vi "Martinas Aging Program v1.0b.vi"() -> ()   [LabVIEW 2011]
uses:
  SubVIs/Control 3.ctl
  <vilib>/ULx/Create Channel.llb/ULx Create Channel (DO-Digital Output).vi
  <vilib>/ULx/Write.llb/ULx Write (Digital U32 1Chan 1Samp).vi
  C:/Program Files (x86)/National Instruments/LabVIEW 2009/instr.lib/Keithley 24XX/Keithley 24XX.lvlib
panel:
  out "Cell Settings Array":T1(array[cluster])=[{"Measure?"=TRUE, "Area (cm^2)"=0.0, "Cell Label"="", "Cell Description"="", "Time between scans (min)"=0.0, "Cell Position"=1, "Scan settings in queue"=0, "Sample holder"=1.0}, {"Measure?"=TRUE, "Area (cm^2)"=0.0, "Cell Label"="", "Cell Description"="", "Time between scans (min)"=0.0, "Cell Position"=2, "Scan settings in queue"=0, "Sample holder"=1.0}, {"Measure?"=TRUE, "Area (cm^2)"=0.0, "Cell Label"="", "Cell Description"="", "Time between scans (min)"=0.0, "Cell Position"=3, "Scan settings in queue"=0, "Sample holder"=1.0}, {"Measure?"=TRUE, "Area (cm^2)"=0.0, "Cell Label"="", "Cell Description"="", "Time between scans (min)"=0.0, "Cell Position"=4, "Scan settings in queue"=0, "Sample holder"=1.0}, {"Measure?"=TRUE, "Area (cm^2)"=0.0, "Cell Label"="", "Cell Description"="", "Time between scans (min)"=0.0, "Cell Position"=5, "Scan settings in queue"=0, "Sample holder"=1.0}, {"Measure?"=TRUE, "Area (cm^2)"=0.0, "Cell Label"="", "Cell Description"="", "Time between scans (min)"=0.0, "Cell Position"=6, "Scan settings in queue"=0, "Sample holder"=1.0}, {"Measure?"=TRUE, "Area (cm^2)"=0.0, "Cell Label"="", "Cell Description"="", "Time between scans (min)"=0.0, "Cell Position"=7, "Scan settings in queue"=0, "Sample holder"=1.0}, {"Measure?"=TRUE, "Area (cm^2)"=0.0, "Cell Label"="", "Cell Description"="", "Time between scans (min)"=0.0, "Cell Position"=8, "Scan settings in queue"=0, "Sample holder"=1.0}, {"Measure?"=TRUE, "Area (cm^2)"=0.0, "Cell Label"="", "Cell Description"="", "Time between scans (min)"=0.0, "Cell Position"=9, "Scan settings in queue"=0, "Sample holder"=1.0}, {"Measure?"=TRUE, "Area (cm^2)"=0.0, "Cell Label"="", "Cell Description"="", "Time between scans (min)"=0.0, "Cell Position"=10, "Scan settings in queue"=0, "Sample holder"=1.0}, {"Measure?"=TRUE, "Area (cm^2)"=0.0, "Cell Label"="", "Cell Description"="", "Time between scans (min)"=0.0, "Cell Position"=11, "Scan settings in queue"=0, "Sample holder"=1.0}, {"Measure?"=TRUE, "Area (cm^2)"=0.0, "Cell Label"="", "Cell Description"="", "Time between scans (min)"=0.0, "Cell Position"=12, "Scan settings in queue"=0, "Sample holder"=1.0}, {"Measure?"=TRUE, "Area (cm^2)"=0.0, "Cell Label"="", "Cell Description"="", "Time between scans (min)"=0.0, "Cell Position"=13, "Scan settings in queue"=0, "Sample holder"=1.0}, {"Measure?"=TRUE, "Area (cm^2)"=0.0, "Cell Label"="", "Cell Description"="", "Time between scans (min)"=0.0, "Cell Position"=14, "Scan settings in queue"=0, "Sample holder"=1.0}, {"Measure?"=TRUE, "Area (cm^2)"=0.0, "Cell Label"="", "Cell Description"="", "Time between scans (min)"=0.0, "Cell Position"=15, "Scan settings in queue"=0, "Sample holder"=1.0}, {"Measure?"=TRUE, "Area (cm^2)"=0.0, "Cell Label"="", "Cell Description"="", "Time between scans (min)"=0.0, "Cell Position"=16, "Scan settings in queue"=0, "Sample holder"=1.0}] {"Scan settings in queue" items=["Regular", "Inverted"]}
  in  "Port":refnum<k21>="Dev0/AuxPort"
  in  "VISA resource name":refnum<visa-resource-name>
  in  "Tab Control":T2(tab)
  in  "Cell Settings Array 1":T3(array[cluster])=[{"Measure?"=TRUE, "Area (cm^2)"=0.0, "Cell Label"="", "Cell Description"="", "Time between scans (s)"=0.0, "Cell Position"=1, "Scan settings in queue"=0, "Sample holder"=1.0}, {"Measure?"=TRUE, "Area (cm^2)"=0.0, "Cell Label"="", "Cell Description"="", "Time between scans (s)"=0.0, "Cell Position"=2, "Scan settings in queue"=0, "Sample holder"=1.0}, {"Measure?"=TRUE, "Area (cm^2)"=0.0, "Cell Label"="", "Cell Description"="", "Time between scans (s)"=0.0, "Cell Position"=3, "Scan settings in queue"=0, "Sample holder"=1.0}, {"Measure?"=TRUE, "Area (cm^2)"=0.0, "Cell Label"="", "Cell Description"="", "Time between scans (s)"=0.0, "Cell Position"=4, "Scan settings in queue"=0, "Sample holder"=1.0}, {"Measure?"=TRUE, "Area (cm^2)"=0.0, "Cell Label"="", "Cell Description"="", "Time between scans (s)"=0.0, "Cell Position"=5, "Scan settings in queue"=0, "Sample holder"=1.0}, {"Measure?"=TRUE, "Area (cm^2)"=0.0, "Cell Label"="", "Cell Description"="", "Time between scans (s)"=0.0, "Cell Position"=6, "Scan settings in queue"=0, "Sample holder"=1.0}, {"Measure?"=TRUE, "Area (cm^2)"=0.0, "Cell Label"="", "Cell Description"="", "Time between scans (s)"=0.0, "Cell Position"=7, "Scan settings in queue"=0, "Sample holder"=1.0}, {"Measure?"=TRUE, "Area (cm^2)"=0.0, "Cell Label"="", "Cell Description"="", "Time between scans (s)"=0.0, "Cell Position"=8, "Scan settings in queue"=0, "Sample holder"=1.0}, {"Measure?"=TRUE, "Area (cm^2)"=0.0, "Cell Label"="", "Cell Description"="", "Time between scans (s)"=0.0, "Cell Position"=9, "Scan settings in queue"=0, "Sample holder"=1.0}, {"Measure?"=TRUE, "Area (cm^2)"=0.0, "Cell Label"="", "Cell Description"="", "Time between scans (s)"=0.0, "Cell Position"=10, "Scan settings in queue"=0, "Sample holder"=1.0}, {"Measure?"=TRUE, "Area (cm^2)"=0.0, "Cell Label"="", "Cell Description"="", "Time between scans (s)"=0.0, "Cell Position"=11, "Scan settings in queue"=0, "Sample holder"=1.0}, {"Measure?"=TRUE, "Area (cm^2)"=0.0, "Cell Label"="", "Cell Description"="", "Time between scans (s)"=0.0, "Cell Position"=12, "Scan settings in queue"=0, "Sample holder"=1.0}, {"Measure?"=TRUE, "Area (cm^2)"=0.0, "Cell Label"="", "Cell Description"="", "Time between scans (s)"=0.0, "Cell Position"=13, "Scan settings in queue"=0, "Sample holder"=1.0}, {"Measure?"=TRUE, "Area (cm^2)"=0.0, "Cell Label"="", "Cell Description"="", "Time between scans (s)"=0.0, "Cell Position"=14, "Scan settings in queue"=0, "Sample holder"=1.0}, {"Measure?"=TRUE, "Area (cm^2)"=0.0, "Cell Label"="", "Cell Description"="", "Time between scans (s)"=0.0, "Cell Position"=15, "Scan settings in queue"=0, "Sample holder"=1.0}, {"Measure?"=TRUE, "Area (cm^2)"=0.0, "Cell Label"="", "Cell Description"="", "Time between scans (s)"=0.0, "Cell Position"=16, "Scan settings in queue"=0, "Sample holder"=1.0}] {"Scan settings in queue" items=["Regular", "Inverted"]}
  in  "Upload from Spreadsheet?":bool
  in  "Upload Spreadsheet path":path
  in  "Save to Spreadsheet?":bool
  in  "Save Spreadsheet Path":path
  in  "Cell Settings Array 2":T1(array[cluster])=[{"Measure?"=TRUE, "Area (cm^2)"=0.0, "Cell Label"="", "Cell Description"="", "Time between scans (min)"=0.0, "Cell Position"=1, "Scan settings in queue"=0, "Sample holder"=2.0}, {"Measure?"=TRUE, "Area (cm^2)"=0.0, "Cell Label"="", "Cell Description"="", "Time between scans (min)"=0.0, "Cell Position"=2, "Scan settings in queue"=0, "Sample holder"=2.0}, {"Measure?"=TRUE, "Area (cm^2)"=0.0, "Cell Label"="", "Cell Description"="", "Time between scans (min)"=0.0, "Cell Position"=3, "Scan settings in queue"=0, "Sample holder"=2.0}, {"Measure?"=TRUE, "Area (cm^2)"=0.0, "Cell Label"="", "Cell Description"="", "Time between scans (min)"=0.0, "Cell Position"=4, "Scan settings in queue"=0, "Sample holder"=2.0}, {"Measure?"=TRUE, "Area (cm^2)"=0.0, "Cell Label"="", "Cell Description"="", "Time between scans (min)"=0.0, "Cell Position"=5, "Scan settings in queue"=0, "Sample holder"=2.0}, {"Measure?"=TRUE, "Area (cm^2)"=0.0, "Cell Label"="", "Cell Description"="", "Time between scans (min)"=0.0, "Cell Position"=6, "Scan settings in queue"=0, "Sample holder"=2.0}, {"Measure?"=TRUE, "Area (cm^2)"=0.0, "Cell Label"="", "Cell Description"="", "Time between scans (min)"=0.0, "Cell Position"=7, "Scan settings in queue"=0, "Sample holder"=2.0}, {"Measure?"=TRUE, "Area (cm^2)"=0.0, "Cell Label"="", "Cell Description"="", "Time between scans (min)"=0.0, "Cell Position"=8, "Scan settings in queue"=0, "Sample holder"=2.0}, {"Measure?"=TRUE, "Area (cm^2)"=0.0, "Cell Label"="", "Cell Description"="", "Time between scans (min)"=0.0, "Cell Position"=9, "Scan settings in queue"=0, "Sample holder"=2.0}, {"Measure?"=TRUE, "Area (cm^2)"=0.0, "Cell Label"="", "Cell Description"="", "Time between scans (min)"=0.0, "Cell Position"=10, "Scan settings in queue"=0, "Sample holder"=2.0}, {"Measure?"=TRUE, "Area (cm^2)"=0.0, "Cell Label"="", "Cell Description"="", "Time between scans (min)"=0.0, "Cell Position"=11, "Scan settings in queue"=0, "Sample holder"=2.0}, {"Measure?"=TRUE, "Area (cm^2)"=0.0, "Cell Label"="", "Cell Description"="", "Time between scans (min)"=0.0, "Cell Position"=12, "Scan settings in queue"=0, "Sample holder"=2.0}, {"Measure?"=TRUE, "Area (cm^2)"=0.0, "Cell Label"="", "Cell Description"="", "Time between scans (min)"=0.0, "Cell Position"=13, "Scan settings in queue"=0, "Sample holder"=2.0}, {"Measure?"=TRUE, "Area (cm^2)"=0.0, "Cell Label"="", "Cell Description"="", "Time between scans (min)"=0.0, "Cell Position"=14, "Scan settings in queue"=0, "Sample holder"=2.0}, {"Measure?"=TRUE, "Area (cm^2)"=0.0, "Cell Label"="", "Cell Description"="", "Time between scans (min)"=0.0, "Cell Position"=15, "Scan settings in queue"=0, "Sample holder"=2.0}, {"Measure?"=TRUE, "Area (cm^2)"=0.0, "Cell Label"="", "Cell Description"="", "Time between scans (min)"=0.0, "Cell Position"=16, "Scan settings in queue"=0, "Sample holder"=2.0}] {"Scan settings in queue" items=["Regular", "Inverted"]}
  in  "Upload Spreadsheet path 2":path
  in  "Upload from Spreadsheet? 2":bool
  in  "Save Spreadsheet Path 2":path
  in  "Save to Spreadsheet?  2":bool
  in  "Cell Settings Array 3":T1(array[cluster])=[{"Measure?"=TRUE, "Area (cm^2)"=0.0, "Cell Label"="", "Cell Description"="", "Time between scans (min)"=0.0, "Cell Position"=1, "Scan settings in queue"=0, "Sample holder"=3.0}, {"Measure?"=TRUE, "Area (cm^2)"=0.0, "Cell Label"="", "Cell Description"="", "Time between scans (min)"=0.0, "Cell Position"=2, "Scan settings in queue"=0, "Sample holder"=3.0}, {"Measure?"=TRUE, "Area (cm^2)"=0.0, "Cell Label"="", "Cell Description"="", "Time between scans (min)"=0.0, "Cell Position"=3, "Scan settings in queue"=0, "Sample holder"=3.0}, {"Measure?"=TRUE, "Area (cm^2)"=0.0, "Cell Label"="", "Cell Description"="", "Time between scans (min)"=0.0, "Cell Position"=4, "Scan settings in queue"=0, "Sample holder"=3.0}, {"Measure?"=TRUE, "Area (cm^2)"=0.0, "Cell Label"="", "Cell Description"="", "Time between scans (min)"=0.0, "Cell Position"=5, "Scan settings in queue"=0, "Sample holder"=3.0}, {"Measure?"=TRUE, "Area (cm^2)"=0.0, "Cell Label"="", "Cell Description"="", "Time between scans (min)"=0.0, "Cell Position"=6, "Scan settings in queue"=0, "Sample holder"=3.0}, {"Measure?"=TRUE, "Area (cm^2)"=0.0, "Cell Label"="", "Cell Description"="", "Time between scans (min)"=0.0, "Cell Position"=7, "Scan settings in queue"=0, "Sample holder"=3.0}, {"Measure?"=TRUE, "Area (cm^2)"=0.0, "Cell Label"="", "Cell Description"="", "Time between scans (min)"=0.0, "Cell Position"=8, "Scan settings in queue"=0, "Sample holder"=3.0}, {"Measure?"=TRUE, "Area (cm^2)"=0.0, "Cell Label"="", "Cell Description"="", "Time between scans (min)"=0.0, "Cell Position"=9, "Scan settings in queue"=0, "Sample holder"=3.0}, {"Measure?"=TRUE, "Area (cm^2)"=0.0, "Cell Label"="", "Cell Description"="", "Time between scans (min)"=0.0, "Cell Position"=10, "Scan settings in queue"=0, "Sample holder"=3.0}, {"Measure?"=TRUE, "Area (cm^2)"=0.0, "Cell Label"="", "Cell Description"="", "Time between scans (min)"=0.0, "Cell Position"=11, "Scan settings in queue"=0, "Sample holder"=3.0}, {"Measure?"=TRUE, "Area (cm^2)"=0.0, "Cell Label"="", "Cell Description"="", "Time between scans (min)"=0.0, "Cell Position"=12, "Scan settings in queue"=0, "Sample holder"=3.0}, {"Measure?"=TRUE, "Area (cm^2)"=0.0, "Cell Label"="", "Cell Description"="", "Time between scans (min)"=0.0, "Cell Position"=13, "Scan settings in queue"=0, "Sample holder"=3.0}, {"Measure?"=TRUE, "Area (cm^2)"=0.0, "Cell Label"="", "Cell Description"="", "Time between scans (min)"=0.0, "Cell Position"=14, "Scan settings in queue"=0, "Sample holder"=3.0}, {"Measure?"=TRUE, "Area (cm^2)"=0.0, "Cell Label"="", "Cell Description"="", "Time between scans (min)"=0.0, "Cell Position"=15, "Scan settings in queue"=0, "Sample holder"=3.0}, {"Measure?"=TRUE, "Area (cm^2)"=0.0, "Cell Label"="", "Cell Description"="", "Time between scans (min)"=0.0, "Cell Position"=16, "Scan settings in queue"=0, "Sample holder"=3.0}] {"Scan settings in queue" items=["Regular", "Inverted"]}
  in  "Upload Spreadsheet path 3":path
  in  "Upload from Spreadsheet? 3":bool
  in  "Save Spreadsheet Path 3":path
  in  "Save to Spreadsheet?  3":bool
  in  "Cell Settings Array 4":T1(array[cluster])=[{"Measure?"=TRUE, "Area (cm^2)"=0.0, "Cell Label"="", "Cell Description"="", "Time between scans (min)"=0.0, "Cell Position"=1, "Scan settings in queue"=0, "Sample holder"=4.0}, {"Measure?"=TRUE, "Area (cm^2)"=0.0, "Cell Label"="", "Cell Description"="", "Time between scans (min)"=0.0, "Cell Position"=2, "Scan settings in queue"=0, "Sample holder"=4.0}, {"Measure?"=TRUE, "Area (cm^2)"=0.0, "Cell Label"="", "Cell Description"="", "Time between scans (min)"=0.0, "Cell Position"=3, "Scan settings in queue"=0, "Sample holder"=4.0}, {"Measure?"=TRUE, "Area (cm^2)"=0.0, "Cell Label"="", "Cell Description"="", "Time between scans (min)"=0.0, "Cell Position"=4, "Scan settings in queue"=0, "Sample holder"=4.0}, {"Measure?"=TRUE, "Area (cm^2)"=0.0, "Cell Label"="", "Cell Description"="", "Time between scans (min)"=0.0, "Cell Position"=5, "Scan settings in queue"=0, "Sample holder"=4.0}, {"Measure?"=TRUE, "Area (cm^2)"=0.0, "Cell Label"="", "Cell Description"="", "Time between scans (min)"=0.0, "Cell Position"=6, "Scan settings in queue"=0, "Sample holder"=4.0}, {"Measure?"=TRUE, "Area (cm^2)"=0.0, "Cell Label"="", "Cell Description"="", "Time between scans (min)"=0.0, "Cell Position"=7, "Scan settings in queue"=0, "Sample holder"=4.0}, {"Measure?"=TRUE, "Area (cm^2)"=0.0, "Cell Label"="", "Cell Description"="", "Time between scans (min)"=0.0, "Cell Position"=8, "Scan settings in queue"=0, "Sample holder"=4.0}, {"Measure?"=TRUE, "Area (cm^2)"=0.0, "Cell Label"="", "Cell Description"="", "Time between scans (min)"=0.0, "Cell Position"=9, "Scan settings in queue"=0, "Sample holder"=4.0}, {"Measure?"=TRUE, "Area (cm^2)"=0.0, "Cell Label"="", "Cell Description"="", "Time between scans (min)"=0.0, "Cell Position"=10, "Scan settings in queue"=0, "Sample holder"=4.0}, {"Measure?"=TRUE, "Area (cm^2)"=0.0, "Cell Label"="", "Cell Description"="", "Time between scans (min)"=0.0, "Cell Position"=11, "Scan settings in queue"=0, "Sample holder"=4.0}, {"Measure?"=TRUE, "Area (cm^2)"=0.0, "Cell Label"="", "Cell Description"="", "Time between scans (min)"=0.0, "Cell Position"=12, "Scan settings in queue"=0, "Sample holder"=4.0}, {"Measure?"=TRUE, "Area (cm^2)"=0.0, "Cell Label"="", "Cell Description"="", "Time between scans (min)"=0.0, "Cell Position"=13, "Scan settings in queue"=0, "Sample holder"=4.0}, {"Measure?"=TRUE, "Area (cm^2)"=0.0, "Cell Label"="", "Cell Description"="", "Time between scans (min)"=0.0, "Cell Position"=14, "Scan settings in queue"=0, "Sample holder"=4.0}, {"Measure?"=TRUE, "Area (cm^2)"=0.0, "Cell Label"="", "Cell Description"="", "Time between scans (min)"=0.0, "Cell Position"=15, "Scan settings in queue"=0, "Sample holder"=4.0}, {"Measure?"=TRUE, "Area (cm^2)"=0.0, "Cell Label"="", "Cell Description"="", "Time between scans (min)"=0.0, "Cell Position"=16, "Scan settings in queue"=0, "Sample holder"=4.0}] {"Scan settings in queue" items=["Regular", "Inverted"]}
  in  "Upload Spreadsheet path 4":path
  in  "Upload from Spreadsheet? 4":bool
  in  "Save Spreadsheet Path 4":path
  in  "Save to Spreadsheet?  4":bool
  out "Table":string[][](table)
  out "JV Curve":cluster{"Y":dbl[], "Y":dbl[]}[](graph)
  in  "Scan Switch":T4=TRUE
  in  "Stop Scan":T4=TRUE
  in  "Upload to the Queue":bool
  in  "Emergency Stop":bool
  in  "Scan settings":u16(ring) items=["Regular", "Inverted"]
  in  "Scan Settings JV":T5={"Light Intensity (Suns)"=1.0, "Stabilization Time (s)"=5.0, "Maximum Voltage (V)"=0.0, "Minimum Voltage (V)"=-1.0, "Range Options"=0, "Scan Direction\nDU (T), UD (F)"=TRUE, "Step Size (V)"=0.01, "Source Delay (s)"=0.15} {"Range Options" items=["Auto Range", "Semi-Auto Range", "100 uA", "1 mA", "10 mA", "100 mA", "1A"]}
  in  "Scan Setting Name":string
  in  "Add to Menu ring":bool
  out "Show me Scan \nSettings JV set":T5={"Light Intensity (Suns)"=1.0, "Stabilization Time (s)"=5.0, "Maximum Voltage (V)"=0.0, "Minimum Voltage (V)"=-1.0, "Range Options"=0, "Scan Direction\nDU (T), UD (F)"=TRUE, "Step Size (V)"=0.01, "Source Delay (s)"=0.15} {"Range Options" items=["Auto Range", "Semi-Auto Range", "100 uA", "1 mA", "10 mA", "100 mA", "1A"]}
  in  "Delete from Menu Ring":bool
  out "TIMER":dbl format="%<%H:%M:%S>t"
  in  "User Set?":bool
  in  "Logout":bool
  in  "Login":bool
  out "Username":string caption="Logged in as:"
  in  "Queue":T6(array[cluster]) {"Scan settings in queue" items=["Regular", "Inverted"]; "Time of the last scan (s)" format="%<%H:%M:%S>t"; "When did you stick it in?" format="%<%H:%M:%S>t"; "Time to next scan (s)" format="%<%H:%M:%S>t"; "Time in rig (s)" format="%<%H:%M:%S>t"}
  # "Area\n(cm^2)"
  # "Time between scans (s)"
  # "Time in rig\n(hrs)"
  # "Time since the last scan (hrs)"
  # "Scan\nnumber"
  # "When did you stick it in?"
  # "Time of the last scan"
  # "Sample\nHolder"
  # "On = working cell\nOff = not working cell"
  # "Label"
  # "Comment"
  # "Cell position"
  # "Scan Settings"
  # "Time between Scans (s)"
  # "Cell\nPosition"
  # "Sample\nHolder"
  # "On = working cell\nOff = not working cell"
  # "Area"
  # "Label"
  # "Comment"
  # "Scan Settings"
  # "Time between Scans (s)"
  # "Cell\nPosition"
  # "Sample\nHolder"
  # "On = working cell\nOff = not working cell"
  # "Area"
  # "Label"
  # "Comment"
  # "Scan Settings"
  # "Time between Scans (s)"
  # "Cell\nPosition"
  # "Sample\nHolder"
  # "On = working cell\nOff = not working cell"
  # "Area"
  # "Label"
  # "Comment"
  # "Scan Settings"
  # "Time between Scans (s)"
  # "Cell\nPosition"
  # "Sample\nHolder"
  # "On = working cell\nOff = not working cell"
  # "Area"
  # "Label"
  # "Comment"
  # "Scan Settings"
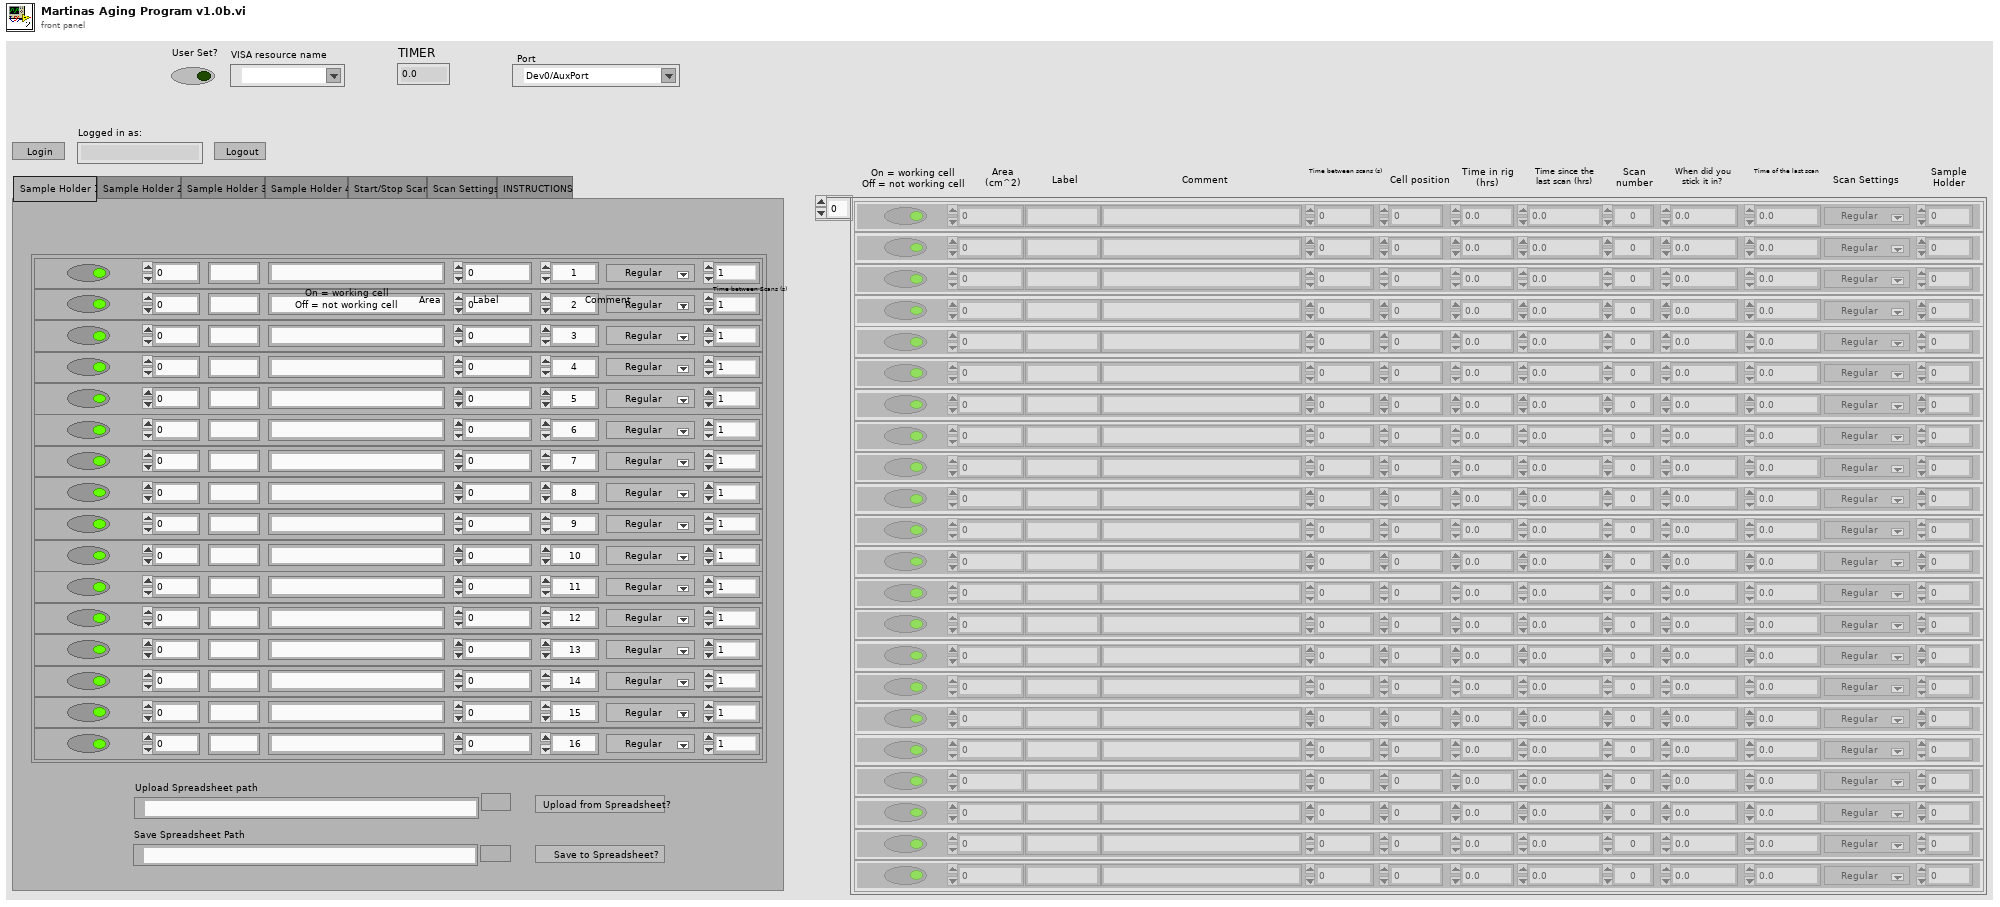
[diagram p1: front panel]
types:
  T1 = cluster{"Measure?":bool, "Area (cm^2)":dbl, "Cell Label":string, "Cell Description":string, "Time between scans (min)":dbl, "Cell Position":i32, "Scan settings in queue":u16, "Sample holder":dbl}[]
  T2 = enum32{"Sample Holder 1", "Sample Holder 2", "Sample Holder 3", "Sample Holder 4", "Start/Stop Scan", "Scan Settings", "INSTRUCTIONS"}
  T3 = cluster{"Measure?":bool, "Area (cm^2)":dbl, "Cell Label":string, "Cell Description":string, "Time between scans (s)":dbl, "Cell Position":i32, "Scan settings in queue":u16, "Sample holder":dbl}[]
  T4 = typedef "Control 3.ctl" = bool
  T5 = cluster{"Light Intensity (Suns)":dbl, "Stabilization Time (s)":dbl, "Maximum Voltage (V)":dbl, "Minimum Voltage (V)":dbl, "Range Options":u16, "Scan Direction\nDU (T), UD (F)":bool, "Step Size (V)":dbl, "Source Delay (s)":dbl}
  T6 = cluster{"Measure?":bool, "Area (cm^2)":dbl, "Cell Label":string, "Cell Description":string, "Cell Position":i32, "Time in rig (s)":dbl, "Time to next scan (s)":dbl, "Scan number":dbl, "When did you stick it in?":dbl, "Time between scans (s)":dbl, "Time of the last scan (s)":dbl, "Scan settings in queue":u16, "Sample Holder":dbl}[]
  T7 = enum8{"Enabled", "Disabled", "Disabled and Grayed Out"}
  T8 = cluster{"Light Intensity (Suns)":dbl, "Stabilization Time (s)":dbl, "Maximum Voltage (V)":dbl, "Minimum Voltage (V)":dbl, "Range Options":u16, "Scan Direction\nDU (T), UD (F)":bool, "Step Size (V)":dbl, "Source Delay (s)":dbl}[]
  T9 = cluster{"Measure?":bool, "Area (cm^2)":dbl, "Cell Label":string, "Cell Description":string, "Cell Position":i32, "Time in rig (s)":dbl, "Time to next scan (s)":dbl, "Scan number":dbl, "When did you stick it in?":dbl, "Time between scans (s)":dbl, "Time of the last scan (s)":dbl, "Scan settings in queue":u16, "Sample Holder":dbl}
  T10 = typedef "imagedata.ctl" = cluster{"image type":i32, "image depth":i32, "image":u8[], "mask":u8[], "colors":u32[], "Rectangle":cluster{"left":i16, "top":i16, "right":i16, "bottom":i16}}
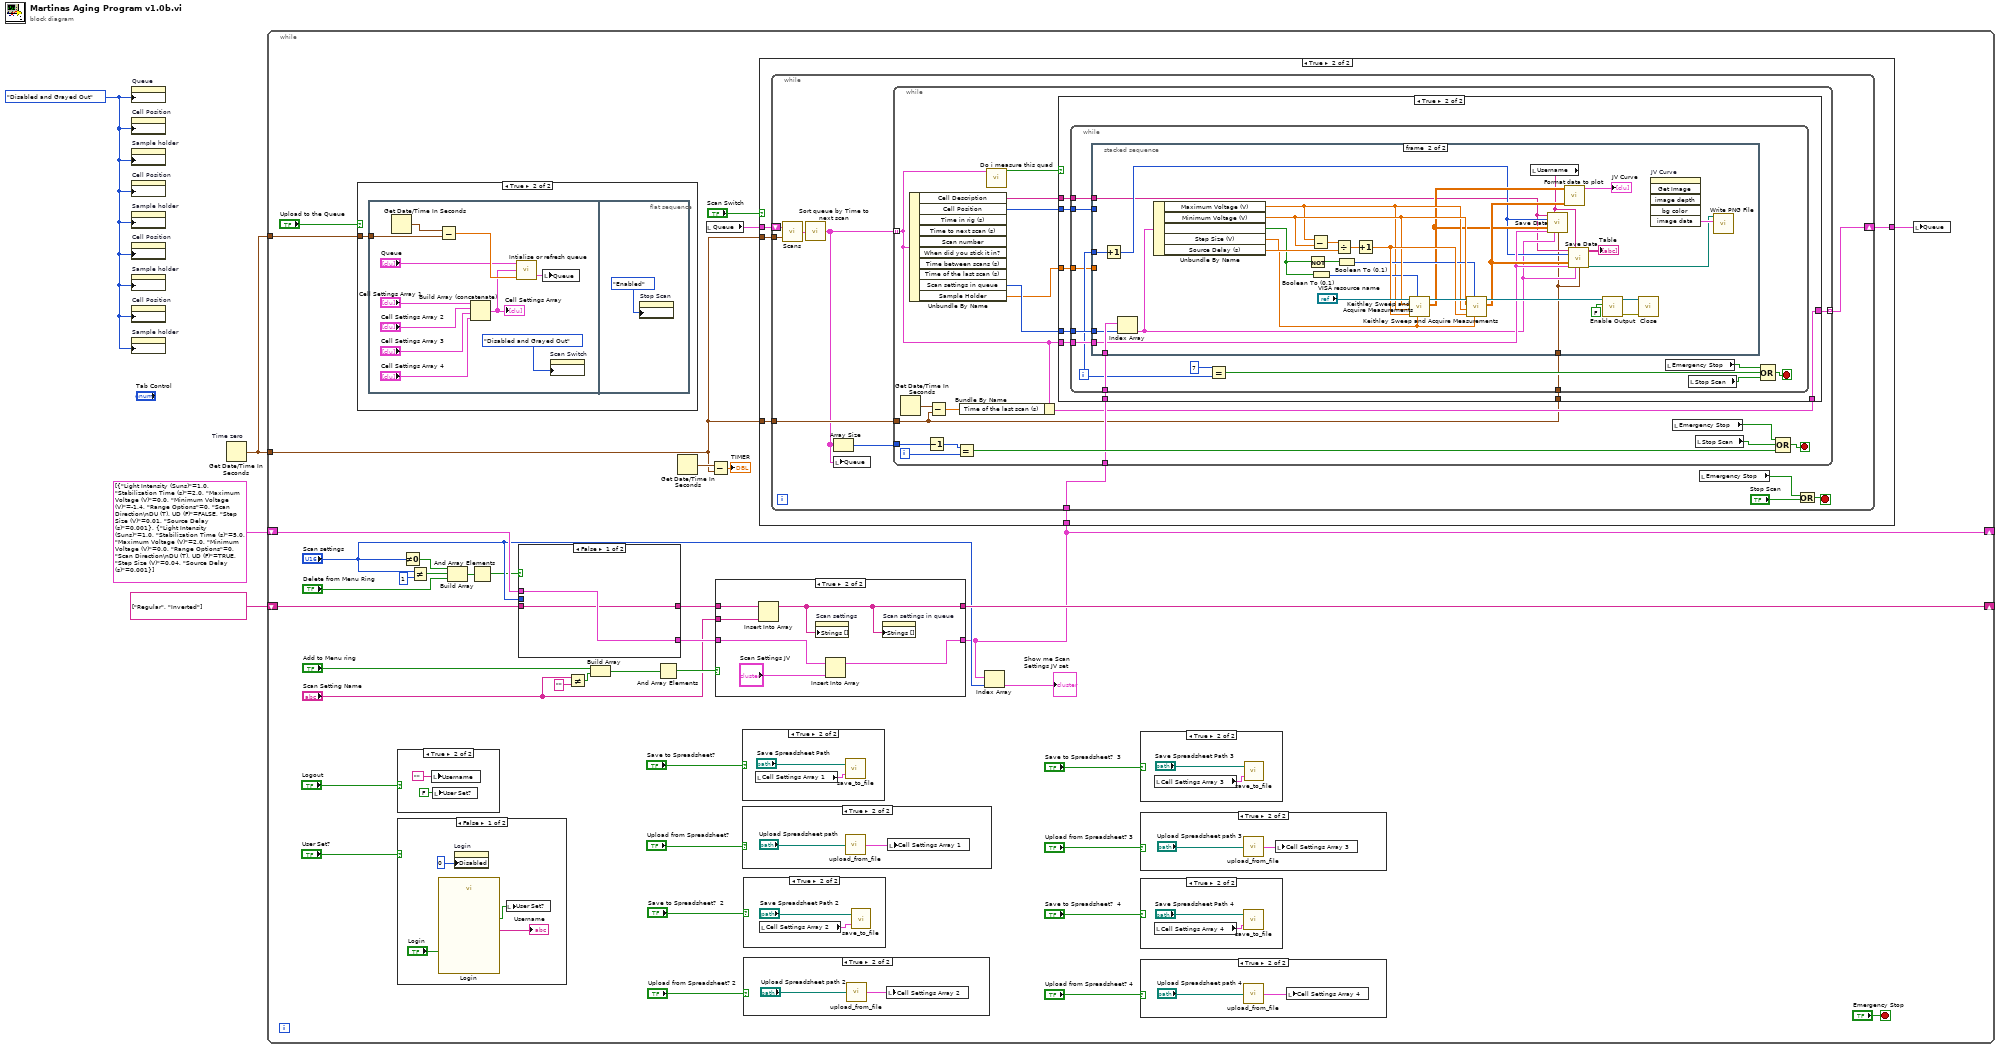
[diagram p0: block diagram]
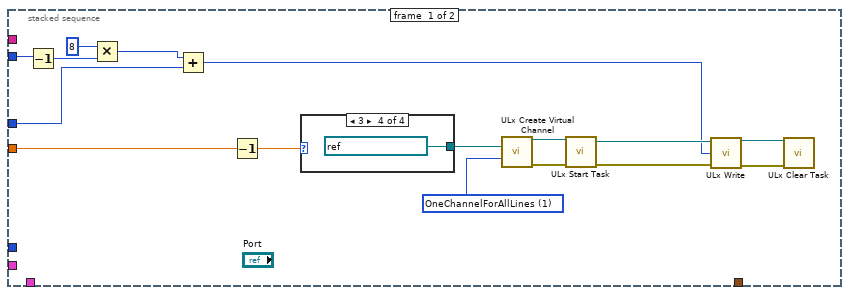
[diagram p10: hidden frame]
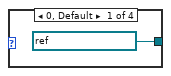
[diagram p11: hidden frame]
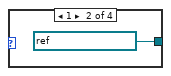
[diagram p12: hidden frame]
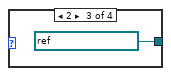
[diagram p13: hidden frame]
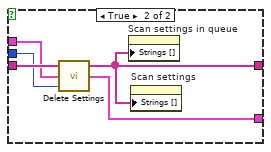
[diagram p14: hidden frame]
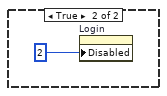
[diagram p17: hidden frame]
diagram:
  w1 = T7."Disabled and Grayed Out" ("Disabled")
  n1 = property on="Queue" class="Arr (strict)"("DisabledEnum"=w1) -> ()  [unwired: 2 in, 2 out]
  n2 = property on="Cell Position" class="DigNum (strict)"("DisabledEnum"=w1) -> ()  [unwired: 2 in, 2 out]
  n3 = property on="Sample holder" class="DigNum (strict)"("DisabledEnum"=w1) -> ()  [unwired: 2 in, 2 out]
  n4 = property on="Cell Position" class="DigNum (strict)"("DisabledEnum"=w1) -> ()  [unwired: 2 in, 2 out]
  n5 = property on="Sample holder" class="DigNum (strict)"("DisabledEnum"=w1) -> ()  [unwired: 2 in, 2 out]
  n6 = property on="Cell Position" class="DigNum (strict)"("DisabledEnum"=w1) -> ()  [unwired: 2 in, 2 out]
  n7 = property on="Sample holder" class="DigNum (strict)"("DisabledEnum"=w1) -> ()  [unwired: 2 in, 2 out]
  n8 = property on="Cell Position" class="DigNum (strict)"("DisabledEnum"=w1) -> ()  [unwired: 2 in, 2 out]
  n9 = property on="Sample holder" class="DigNum (strict)"("DisabledEnum"=w1) -> ()  [unwired: 2 in, 2 out]
  n10 = Get Date/Time In Seconds "Time zero"() -> (seconds since 1Jan1904=w2:timestamp)
  n11 = while {
    tunnel: w2 -> [w40]
    shift-right: [w7] -> _
    shift-left: T8 [{"Light Intensity (Suns)"=1.0, "Stabilization Time (s)"=2.0, "Maximum Voltage (V)"=0.0, "Minimum Voltage (V)"=-1.4, "Range Options"=0, "Scan Direction\nDU (T), UD (F)"=FALSE, "Step Size (V)"=0.01, "Source Delay (s)"=0.001}, {"Light Intensity (Suns)"=1.0, "Stabilization Time (s)"=5.0, "Maximum Voltage (V)"=2.0, "Minimum Voltage (V)"=0.0, "Range Options"=0, "Scan Direction\nDU (T), UD (F)"=TRUE, "Step Size (V)"=0.04, "Source Delay (s)"=0.001}] ("JV curve scan settings 2") -> [w34]
    shift-right: [w38] -> _
    shift-left: string[] ["Regular", "Inverted"] ("Strings []") -> [w35]
    tunnel: w2 -> [w6]
    stop <- "Emergency Stop" stop-if-true
    n12 = case shown="True" "Upload to the Queue" {
      tunnel: w40 -> [_ w188]
      frame False {
      }
      frame True {
        n13 = flat-sequence {
          tunnel: w188 -> [w199]
          frame #0 {
            n14 = Get Date/Time In Seconds() -> (seconds since 1Jan1904=w198:timestamp)
            n15 = Subtract(x=w198, y=w199) -> (x-y=w197:dbl)
            n16 = Build Array (concatenate)("Cell Settings Array 1", "Cell Settings Array 2", "Cell Settings Array 3", "Cell Settings Array 4") -> (w190:T1)
            "Cell Settings Array" <- w190
            n17 = call "Intialise or refresh queue.vi"("When did you stick it in?"=w197, "Cell Settings Array"=w190, "Queue in"="Queue") -> ("Queue out"=w196:T6)  [unwired: 1 in]
            n18 = local write "Queue"(w196) -> ()
            n19 = property on="Scan Switch" class="Bool (strict)"("DisabledEnum"=T7."Disabled and Grayed Out" ("Disabled")) -> ()  [unwired: 2 in, 2 out]
          }
          frame #1 {
            n20 = property on="Stop Scan" class="Bool (strict)"("DisabledEnum"=T7."Enabled" ("Disabled")) -> ()  [unwired: 2 in, 2 out]
          }
        }
      }
    }
    n21 = case shown="True" "Logout" {
      frame False {
      }
      frame True {
        n22 = local write "Username"("") -> ()
        n23 = local write "User Set?"(FALSE) -> ()
      }
    }
    n24 = case shown="False" "User Set?" {
      frame False {
        n25 = call "Login"("Enable"="Login") -> ("Username"=→"Username":string, "OK"=w183:bool)  [unwired: 16 in, 1 out]
        n26 = property on="Login" class="Bool"("Disabled"=0) -> ()  [unwired: 2 in, 2 out]
        n27 = local write "User Set?"(w183) -> ()
      }
      frame True {
        n28 = property on="Login" class="Bool"("Disabled"=2) -> ()  [unwired: 2 in, 2 out]
      }
    }
    n29 = Not Equal To 0?(x="Scan settings") -> (x != 0?=w31:bool)
    n30 = Not Equal?(x="Scan settings", y=u16 1) -> (x != y?=w28:bool)
    n31 = Build Array(w31, w28, "Delete from Menu Ring") -> (w26:bool[])
    n32 = And Array Elements(Boolean array=w26) -> (logical AND=w25:bool)
    n33 = case shown="False" w25 {
      tunnel: w35 -> [w166 w172]
      tunnel: w34 -> [w167 w171]
      tunnel: "Scan settings" -> [_ w170]
      tunnel: [w166 w169] -> w33
      tunnel: [w167 w168] -> w32
      frame False {
      }
      frame True {
        n34 = call "Delete Settings.vi"("Scan settings"=w170, "JV curve scan settings"=w171, "Strings In"=w172) -> ("JV curve scan settings Out"=w168:T8, "Strings Out"=w169:string[])  [unwired: 1 out]
        n35 = property on="Scan settings in queue" class="Ring (strict)"("Strings []"=w169) -> ()  [unwired: 2 in, 2 out]
        n36 = property on="Scan settings" class="Ring (strict)"("Strings []"=w169) -> ()  [unwired: 2 in, 2 out]
      }
    }
    n37 = Not Equal?(x="Scan Setting Name", y="") -> (x != y?=w22:bool)
    n38 = Build Array("Add to Menu ring", w22) -> (w23:bool[])
    n39 = And Array Elements(Boolean array=w23) -> (logical AND=w20:bool)
    n40 = Get Date/Time In Seconds() -> (seconds since 1Jan1904=w17:timestamp)
    n41 = local read "Queue"() -> (w15:T6)
    n42 = Subtract(x=w17, y=w6) -> (x-y=→"TIMER":dbl)
    n43 = case shown="True" w20 {
      tunnel: w32 -> [w174 w180]
      tunnel: [w174 w179] -> w7
      tunnel: w33 -> [w173 w176]
      tunnel: [w173 w177] -> w38
      tunnel: "Scan Setting Name" -> [_ w175]
      frame False {
      }
      frame True {
        n44 = Insert Into Array(array=w176, new element=w175) -> (w177:string[])  [unwired: 1 in]
        n45 = property on="Scan settings" class="Ring (strict)"("Strings []"=w177) -> ()  [unwired: 2 in, 2 out]
        n46 = Insert Into Array(array=w180, new element="Scan Settings JV") -> (w179:T8)  [unwired: 1 in]
        n47 = property on="Scan settings in queue" class="Ring (strict)"("Strings []"=w177) -> ()  [unwired: 2 in, 2 out]
      }
    }
    n48 = case shown="True" "Save to Spreadsheet?" {
      frame False {
      }
      frame True {
        n49 = local read "Cell Settings Array 1"() -> (w201:T3)
        n50 = call "save_to_file.vi"("Cell Settings Array 4"=w201, "Save Path"="Save Spreadsheet Path") -> ()  [unwired: 1 in]
      }
    }
    n51 = case shown="True" "Upload from Spreadsheet?" {
      frame False {
      }
      frame True {
        n52 = call "upload_from_file.vi"("Spreadsheet path"="Upload Spreadsheet path") -> ("Cell Settings Array 4"=w203:T1)
        n53 = local write "Cell Settings Array 1"(w203) -> ()
      }
    }
    n54 = case shown="True" "Save to Spreadsheet?  2" {
      frame False {
      }
      frame True {
        n55 = local read "Cell Settings Array 2"() -> (w52:T1)
        n56 = call "save_to_file.vi"("Cell Settings Array 4"=w52, "Save Path"="Save Spreadsheet Path 2") -> ()  [unwired: 1 in]
      }
    }
    n57 = case shown="True" "Upload from Spreadsheet? 2" {
      frame False {
      }
      frame True {
        n58 = call "upload_from_file.vi"("Spreadsheet path"="Upload Spreadsheet path 2") -> ("Cell Settings Array 4"=w54:T1)
        n59 = local write "Cell Settings Array 2"(w54) -> ()
      }
    }
    n60 = case shown="True" "Scan Switch" {
      tunnel: w15 -> [w56 w61]
      tunnel: w6 -> [_ w60]
      tunnel: [w56 w58] -> w5
      tunnel: w7 -> [_ w59]
      tunnel: w6 -> [_ w57]
      frame False {
      }
      frame True {
        n61 = while {
          tunnel: w60 -> [w71]
          tunnel: w59 -> [w69]
          shift-right: [w67] -> w58
          shift-left: w61 -> [w72]
          tunnel: w57 -> [w66]
          stop <- w64 stop-if-true
          n62 = call "Scans.vi"("Time zero (sec)"=w71, "Queue in"=w72) -> ("Queue out"=w70:T6)
          n63 = call "Sort queue by Time to next scan.vi"("Queue"=w70) -> ("Queue Out"=w65:T6)  [unwired: 4 in]
          n64 = Array Size(array=w65) -> (size(s)=w68:i32)
          n65 = local write "Queue"(w65) -> ()
          n66 = while {
            tunnel: w65 -> [w76] mode=indexing
            tunnel: w69 -> [w82]
            tunnel: w68 -> [w88]
            tunnel: [w83] -> w67 mode=indexing
            tunnel: w66 -> [w74]
            i -> [w90]
            stop <- w86 stop-if-true
            n67 = Get Date/Time In Seconds() -> (seconds since 1Jan1904=w78:timestamp)
            n68 = Unbundle By Name(w76) -> ("Cell Description"=w80:string, "Cell Position"=w84:i32, "Scan settings in queue"=w91:u16, "Sample Holder"=w81:dbl)  [unwired: 6 out]
            n69 = Decrement(x=w88) -> (x-1=w89:i32)
            n70 = Subtract(x=w78, y=w74) -> (x-y=w77:dbl)
            n71 = Equal?(x=w89, y=w90) -> (x = y?=w87:bool)
            n72 = Bundle By Name(cluster=w76, "Time of the last scan (s)"=w77) -> (w75:T9)
            n73 = call "Do i measure this quad.vi"("Cell details"=w76) -> ("Measure cell?"=w79:bool)  [unwired: 10 in]
            n74 = case shown="True" w79 {
              tunnel: w82 -> [_ w100]
              tunnel: w91 -> [_ w99]
              tunnel: w76 -> [w92 w98]
              tunnel: w84 -> [_ w97]
              tunnel: [w92 w94] -> w83
              tunnel: w81 -> [_ w96]
              tunnel: w80 -> [_ w95]
              tunnel: w75 -> [_ w94]
              tunnel: w74 -> [_ w93]
              frame False {
              }
              frame True {
                n75 = while {
                  tunnel: w100 -> [w113]
                  tunnel: w99 -> [w112]
                  tunnel: w98 -> [w111]
                  tunnel: w97 -> [w110]
                  tunnel: w96 -> [w104]
                  tunnel: w95 -> [w103]
                  tunnel: w93 -> [w102]
                  i -> [w105]
                  stop <- w107 stop-if-true
                  n76 = stacked-sequence {
                    tunnel: w113 -> [_ w161]
                    tunnel: w112 -> [_ w160]
                    tunnel: w111 -> [_ w141]
                    tunnel: w110 -> [w118 _]
                    tunnel: w105 -> [w115 w139]
                    tunnel: w104 -> [w114 _]
                    tunnel: w103 -> [_ w135]
                    tunnel: w102 -> [_ w134]
                    frame #0 {
                      w127 = 1 items=["OneChannelForEachLine", "OneChannelForAllLines"] ("line grouping")
                      n77 = Decrement(x=w118) -> (x-1=w117:i32)
                      n78 = Multiply(x=8, y=w117) -> (x*y=w119:i32)
                      n79 = Add(x=w119, y=w115) -> (x+y=w116:i32)
                      n80 = Decrement(x=w114) -> (x-1=w128:dbl)
                      n81 = case shown="3" w128 {
                        tunnel: [refnum<k21> "Dev0/1stPortA" ("Port 2") refnum<k21> "Dev0/1stPortB" ("Port 2") refnum<k21> "Dev0/1stPortA" ("Port 2") refnum<k21> "Dev0/1stPortB" ("Port 2")] -> w129
                        frame 0, Default {
                        }
                        frame 1 {
                        }
                        frame 2 {
                        }
                        frame 3 {
                        }
                      }
                      n82 = call-poly <vilib>:"ULx Create Virtual Channel.vi"("lines"=w129, "line grouping"=w127) -> ("task out"=w125:refnum<k24>, "error out"=w126:errorcluster)  [unwired: 12 in]
                      n83 = call <vilib>:"ULx Start Task.vi"("task in"=w125, "error in"=w126) -> ("task out"=w122:refnum<k24>, "error out"=w121:errorcluster)  [unwired: 12 in]
                      n84 = call-poly <vilib>:"ULx Write.vi"("task in"=w122, "data"=w116, "error in"=w121) -> ("task out"=w124:refnum<k24>, "error out"=w123:errorcluster)  [unwired: 10 in, 1 out]
                      n85 = call <vilib>:"ULx Clear Task.vi"("task in"=w124, "error in"=w123) -> ()  [unwired: 13 in, 1 out]
                    }
                    frame #1 {
                      n86 = Increment(x=w139) -> (x+1=w138:i32)
                      n87 = Index Array(array=w161, index=w160) -> (element=w137:T5)
                      n88 = Unbundle By Name(w137) -> ("Maximum Voltage (V)"=w147:dbl, "Minimum Voltage (V)"=w153:dbl, "Scan Direction\nDU (T), UD (F)"=w151:bool, "Step Size (V)"=w157:dbl, "Source Delay (s)"=w148:dbl)
                      n89 = Not(x=w151) -> (.not. x?=w152:bool)
                      n90 = Subtract(x=w147, y=w153) -> (x-y=w158:dbl)
                      n91 = Boolean To (0,1)(Boolean=w151) -> (0, 1=w149:i16)
                      n92 = Divide(x=w158, y=w157) -> (x/y=w159:dbl)
                      n93 = Boolean To (0,1)(Boolean=w152) -> (0, 1=w150:i16)
                      n94 = Increment(x=w159) -> (x+1=w155:dbl)
                      n95 = call "Keithley Sweep and Acquire Measurements.vi"("Source Delay (s)"=w148, "Sweep Direction"=w149, "Number of Points"=w155, "Maximum Amplitude"=w147, "Minimum Amplitude"=w153, "VISA resource name"="VISA resource name") -> ("Data Array"=w140:dbl[][], "VISA resource name out"=w156:refnum<visa-resource-name>)  [unwired: 1 in, 1 out]
                      n96 = call "Keithley Sweep and Acquire Measurements.vi"("Source Delay (s)"=w148, "Sweep Direction"=w150, "Number of Points"=w155, "Maximum Amplitude"=w147, "Minimum Amplitude"=w153, "VISA resource name"=w156) -> ("Data Array"=w143:dbl[][], "VISA resource name out"=w154:refnum<visa-resource-name>)  [unwired: 1 in, 1 out]
                      n97 = local read "Username"() -> (w136:string)
                      n98 = call "Save Data.vi"("Experiment Indicator"=w135, "Username"=w136, "Pixel"=w138, "Data Array"=w140, "Cell details cluster"=w141, "Show me Scan \nSettings JV set"=w137, "Time zero"=w134) -> ()  [unwired: 4 in, 5 out]
                      n99 = call "Format data to plot.vi"("Data Array 2"=w143, "Data Array"=w140) -> ("JV Curve"=→"JV Curve":cluster{"Y":dbl[], "Y":dbl[]}[])  [unwired: 9 in]
                      n100 = call "Save Data.vi"("Experiment Indicator"=w135, "Username"=w136, "Pixel"=w138, "Data Array"=w143, "Cell details cluster"=w141, "Show me Scan \nSettings JV set"=w137, "Time zero"=w134) -> ("Master Log"=→"Table":string[][], "File path for JV image"=w142:path)  [unwired: 4 in, 3 out]
                      n101 = call "Enable Output.vi"("Enable Output (T: Enable)"=FALSE, "VISA resource name"=w154) -> ("error out"=w164:errorcluster, "VISA resource name out"=w165:refnum<visa-resource-name>)  [unwired: 8 in]
                      n102 = call "Close.vi"("error in (no error)"=w164, "VISA resource name"=w165) -> ()  [unwired: 9 in, 1 out]
                      n103 = invoke on="JV Curve" class="XYGraph (strict)" method="Get Image"() -> ("image data"=w145:T10)  [unwired: 6 in, 5 out]
                      n104 = call <vilib>:"Write PNG File.vi"("image data"=w145, "path to PNG file"=w142) -> ()  [unwired: 8 in, 2 out]
                    }
                  }
                  n105 = Equal?(x=7, y=w105) -> (x = y?=w106:bool)
                  n106 = local read "Emergency Stop"() -> (w101:bool)
                  n107 = local read "Stop Scan"() -> (w108:T4)
                  n108 = Compound Arithmetic op=OR(w101, w106, w108) -> (w107:T4)
                }
              }
            }
            n109 = local read "Emergency Stop"() -> (w73:bool)
            n110 = local read "Stop Scan"() -> (w85:T4)
            n111 = Compound Arithmetic op=OR(w73, w85, w87) -> (w86:T4)
          }
          n112 = local read "Emergency Stop"() -> (w62:bool)
          n113 = Or(x=w62, y="Stop Scan") -> (x .or. y?=w64:T4)
        }
      }
    }
    n114 = Index Array(array=w7, index="Scan settings") -> (element=→"Show me Scan \nSettings JV set":T5)
    n115 = case shown="True" "Save to Spreadsheet?  3" {
      frame False {
      }
      frame True {
        n116 = local read "Cell Settings Array 3"() -> (w48:T1)
        n117 = call "save_to_file.vi"("Cell Settings Array 4"=w48, "Save Path"="Save Spreadsheet Path 3") -> ()  [unwired: 1 in]
      }
    }
    n118 = case shown="True" "Upload from Spreadsheet? 3" {
      frame False {
      }
      frame True {
        n119 = call "upload_from_file.vi"("Spreadsheet path"="Upload Spreadsheet path 3") -> ("Cell Settings Array 4"=w50:T1)
        n120 = local write "Cell Settings Array 3"(w50) -> ()
      }
    }
    n121 = case shown="True" "Save to Spreadsheet?  4" {
      frame False {
      }
      frame True {
        n122 = local read "Cell Settings Array 4"() -> (w44:T1)
        n123 = call "save_to_file.vi"("Cell Settings Array 4"=w44, "Save Path"="Save Spreadsheet Path 4") -> ()  [unwired: 1 in]
      }
    }
    n124 = case shown="True" "Upload from Spreadsheet? 4" {
      frame False {
      }
      frame True {
        n125 = call "upload_from_file.vi"("Spreadsheet path"="Upload Spreadsheet path 4") -> ("Cell Settings Array 4"=w46:T1)
        n126 = local write "Cell Settings Array 4"(w46) -> ()
      }
    }
    n127 = local write "Queue"(w5) -> ()
  }
